vi "Read_N_Args.vi"(6 "Delay (ms)":u32=5000, 8 "Error IN":errorcluster, 9 "Nb_Args":i32=1, 10 "Arg_Char":string="\r", 11 "VRN IN":refnum<visa-resource-name>) -> (0 "Error OUT":errorcluster, 1 "All_Args?":bool, 2 "Answer":string, 3 "VRN OUT":refnum<visa-resource-name>)   [LabVIEW 2011]
panel:
  out "ExecTime":u32
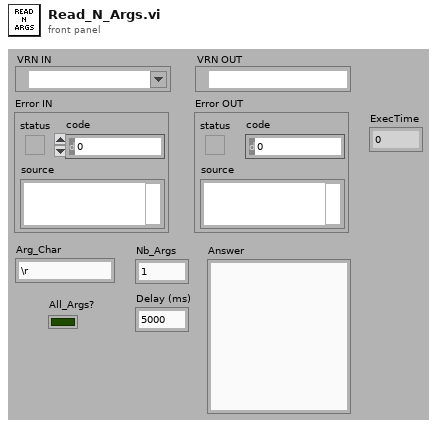
[diagram p1: front panel]
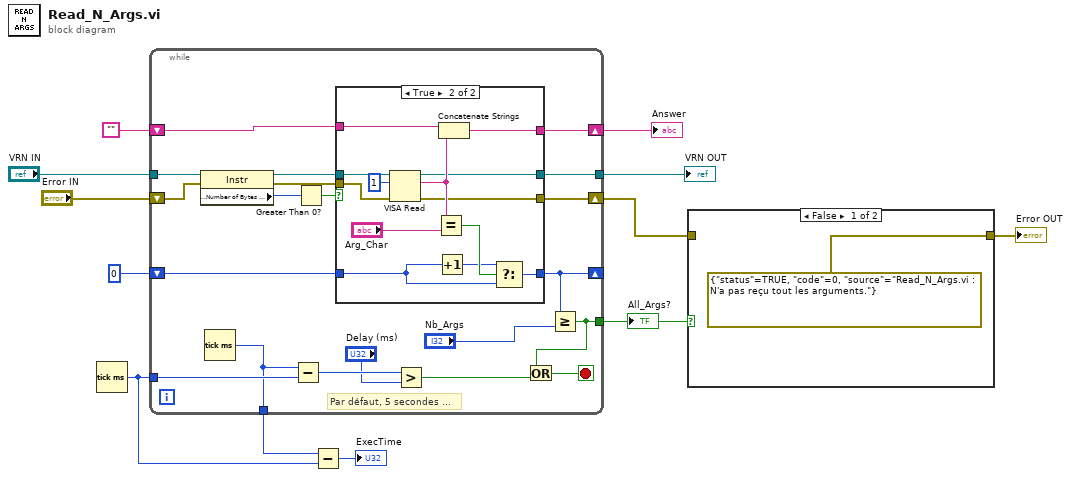
[diagram p0: block diagram]
diagram:
  n1 = Tick Count (ms)() -> (millisecond timer value=w2:u32)
  n2 = while {
    tunnel: "VRN IN" -> [w27]
    tunnel: w2 -> [w32]
    shift-right: [w20] -> w7
    shift-left: "" -> [w23]
    shift-right: [w18] -> _
    shift-left: 0 -> [w19]
    shift-right: [w16] -> w6
    shift-left: "Error IN" -> [w26]
    tunnel: [w15] -> w4
    tunnel: [w14] -> w10
    tunnel: [w13] -> w3
    stop <- w30 stop-if-true
    # "Par défaut, 5 secondes ..."
    n3 = property class="Instr"(reference=w27, error in=w26) -> (reference out=w22:refnum<visa-resource-name>, error out=w21:errorcluster, "Serial Settings:Number of Bytes at Serial Port"=w25:u32)
    n4 = Tick Count (ms)() -> (millisecond timer value=w13:u32)
    n5 = Subtract(x=w13, y=w32) -> (x-y=w31:u32)
    n6 = Greater Than 0?(x=w25) -> (x > 0?=w24:bool)
    n7 = case shown="True" w24 {
      tunnel: w23 -> [w36 w47]
      tunnel: w22 -> [w33 w49]
      tunnel: w21 -> [w34 w48]
      tunnel: [w36 w46] -> w20
      tunnel: w19 -> [w35 w41]
      tunnel: [w35 w43] -> w18
      tunnel: [w34 w40] -> w16
      tunnel: [w33 w39] -> w14
      frame False {
      }
      frame True {
        n8 = VISA Read(VISA resource name=w49, byte count=u32 1, error in (no error)=w48) -> (VISA resource name out=w39:refnum<visa-resource-name>, read buffer=w45:string, error out=w40:errorcluster)  [unwired: 1 out]
        n9 = Equal?(x=w45, y="Arg_Char") -> (x = y?=w44:bool)
        n10 = Increment(x=w41) -> (x+1=w42:i32)
        n11 = Concatenate Strings(w47, w45) -> (w46:string)
        n12 = Select(t=w42, s=w44, f=w41) -> (s? t:f=w43:i32)
      }
    }
    n13 = Greater?(x=w31, y="Delay (ms)") -> (0:w29:bool)
    n14 = Greater Or Equal?(x=w18, y="Nb_Args") -> (x >= y?=w15:bool)
    n15 = Or(x=w15, y=w29) -> (x .or. y?=w30:bool)
  }
  "VRN OUT" <- w10
  "Answer" <- w7
  "All_Args?" <- w4
  n16 = Subtract(x=w3, y=w2) -> (x-y=→"ExecTime":u32)
  n17 = case shown="False" w4 {
    tunnel: w6 -> [_ w51]
    tunnel: [errorcluster {"status"=TRUE, "code"=0, "source"="Read_N_Args.vi : N'a pas reçu tout les arguments."} ("Error IN") w51] -> w5
    frame False {
    }
    frame True {
    }
  }
  "Error OUT" <- w5
